vi "Auto Mute.vi"(8 "Error In":errorcluster, 10 "Auto Mute":bool, 11 "KIT-QVA in":refnum<class "KIT-QVA.lvclass">) -> (0 "Error Out":errorcluster, 3 "KIT-QVA out":refnum<class "KIT-QVA.lvclass">)   [LabVIEW 2015, in "KIT-QVA.lvlib" / "KIT-QVA.lvclass"]
doc: "Activate automatic, time limited, detector muting."
uses:
  KIT-QVA.lvclass
  KIT-QVA.lvclass/KIT-QVA.ctl
  instr.lib/KIT-QV/KIT QV.lvlib
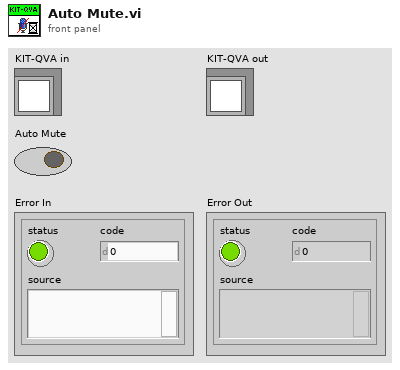
[diagram p1: front panel]
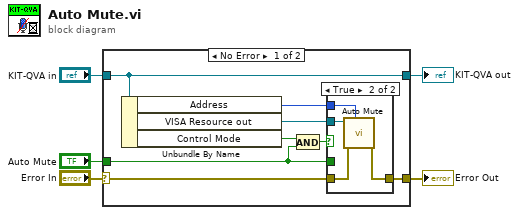
[diagram p0: block diagram]
diagram:
  n1 = case shown="No Error" "Error In" {
    selector: "Error In" -> [w10 w20]
    tunnel: [w9 w20] -> w4
    tunnel: [w13 w19] -> w2
    tunnel: "KIT-QVA in" -> [w13 w19]
    tunnel: "Auto Mute" -> [w6 _]
    frame No Error {
      n2 = Unbundle By Name(w13) -> ("Address"=w11:u16, "VISA Resource out"=w12:refnum<visa-resource-name>, "Control Mode"=w8:bool)
      n3 = And(x=w8, y=w6) -> (x .and. y?=w7:bool)
      n4 = case shown="True" w7 {
        tunnel: w12 -> [_ w16]
        tunnel: w11 -> [_ w15]
        tunnel: w10 -> [w14 w18]
        tunnel: w6 -> [_ _]
        tunnel: [w14 w17] -> w9
        frame False {
        }
        frame True {
          n5 = call "Auto Mute.vi"("Address"=w15, "Error In"=w18, "VISA Resource in"=w16) -> ("Error Out"=w17:errorcluster)  [unwired: 7 in, 1 out]
        }
      }
    }
    frame Error {
    }
  }
  "Error Out" <- w4
  "KIT-QVA out" <- w2
